vi "BEEP.vi"() -> ()   [LabVIEW 2020]
uses:
  Windows/System32/kernel32.dll
panel:
  out "sortie d'erreur":errorcluster
  out "type de retour":i32
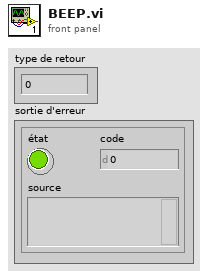
[diagram p1: front panel]
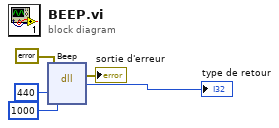
[diagram p0: block diagram]
diagram:
  n1 = dll-call lib="C:/Windows/System32/kernel32.dll" fn="Beep"(error in=errorcluster {"status"=FALSE, "code"=0, "source"=""} ("entrée d'erreur (pas d'erreur)"), "freq"=440, "duree"=1000) -> (error out=→"sortie d'erreur":errorcluster, "type de retour"=→"type de retour":i32)  [unwired: 4 in, 1 out]
